vi "Do.vi"(8 "error in":errorcluster, 10 "Actor in":refnum<class "Actor.lvclass">, 11 "Send External Stop MSG":refnum<class "Send External Stop MSG.lvclass">) -> (0 "error out":errorcluster, 2 "Actor out":refnum<class "Actor.lvclass">)   [LabVIEW 2014, in "Calibration.lvlib" / "Send External Stop MSG.lvclass"]
doc: "(<B>Filename</B>: Actor Framework.lvlib:Message.lvclass:Do.vi)\n\nDefines what a message does when it is received by an actor. Generally, a message instructs an actor to invoke one of its methods. By default, this method does nothing. A child class must override it to define behavior. Create a child class by using the Actor Framework Message Maker dialog box."
uses:
  Send External Stop MSG.lvclass
  <vilib>/ActorFramework/Actor/Actor.lvclass
  Actor/Calibration Actor.lvclass
  Actor/Calibration Actor.lvclass/Calibration Actor.ctl
  SuperActor/SuperActor.lvclass/SuperActor.ctl
  Actor/Read ext_stop.vi
  SuperActor/Read Log Session.vi
  <userlib>/_Session Fwk/Session - Root.lvclass
  reusable/Session APIs/Session Log/System Log.lvclass
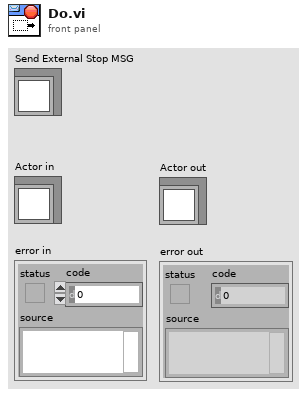
[diagram p1: front panel]
types:
  T1 = typedef "Session - Root.lvclass/Session Handle.ctl" = refnum<data-value>
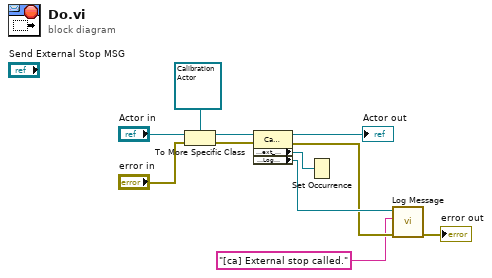
[diagram p0: block diagram]
diagram:
  n1 = To More Specific Class(target class=refnum<class "Calibration Actor.lvclass"> refnum ("Calibration.lvlib:Calibration Actor"), reference="Actor in", error in="error in") -> (specific class reference=w8:refnum<class "Calibration Actor.lvclass">, error out=w7:errorcluster)
  n2 = property class="Calibration Actor"(reference=w8, error in=w7) -> (reference out=→"Actor out":refnum<class "Calibration Actor.lvclass">, error out=w3:errorcluster, "Accessors:ext_stop"=w5:refnum<k4>, "Accessors:Log Session"=w4:T1)
  n3 = Set Occurrence(w5) -> ()
  n4 = call "Log Message.vi"("error in"=w3, "MSG In"="[ca] External stop called.", "session in"=w4) -> ("error out"=→"error out":errorcluster)  [unwired: 7 in, 1 out]
